vi "Adv_Deregister_for_Callback.vi"(8 "error in (no error)":errorcluster, 11 "LightField Automation in":refnum<class "LightField Automation.lvclass">) -> (0 "error out":errorcluster, 3 "LightField Automation out":refnum<class "LightField Automation.lvclass">)   [LabVIEW 2013, in "LightField Automation.lvclass"]
uses:
  LightField Automation.lvclass
  LightField Automation.lvclass/LightField Automation.ctl
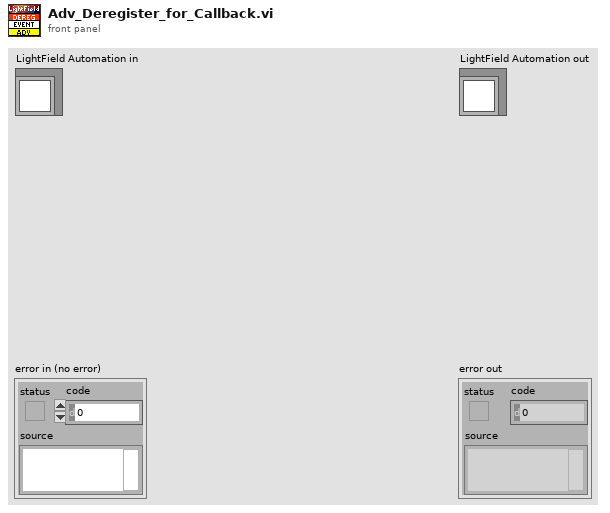
[diagram p1: front panel]
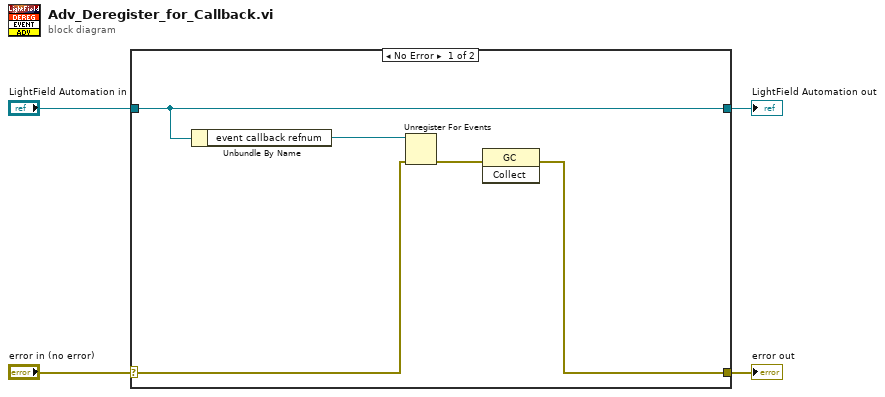
[diagram p0: block diagram]
diagram:
  n1 = case shown="No Error" "error in (no error)" {
    selector: "error in (no error)" -> [w8 w11]
    tunnel: [w5 w11] -> w3
    tunnel: [w9 w10] -> w1
    tunnel: "LightField Automation in" -> [w9 w10]
    frame No Error {
      n2 = Unbundle By Name(w9) -> ("event callback refnum"=w7:refnum<k27>)
      n3 = Unregister For Events(event registration refnum=w7, error in=w8) -> (error out=w6:errorcluster)
      n4 = invoke class="GC" method="Collect"(error in=w6) -> (error out=w5:errorcluster)  [unwired: 2 in, 2 out]
    }
    frame Error {
    }
  }
  "error out" <- w3
  "LightField Automation out" <- w1
